vi "Update Control Board.vi"(8 "error in (no error)":errorcluster, 9 "PWM Outputs":T3, 10 "LED Outputs":T4, 11 "Control Board VISA Reference In":refnum<visa-resource-name>) -> (0 "error out":errorcluster, 1 "Analog Inputs":T2, 2 "Switch Inputs":T1, 3 "Control Board VISA Reference Out":refnum<visa-resource-name>, 4 "CRC Status":bool)   [LabVIEW 2013]
uses:
  LED_Output_TypeDef.ctl
  PWM_Output_TypeDef.ctl
  Analog_Input_TypeDef.ctl
  Switch_Input_TypeDef.ctl
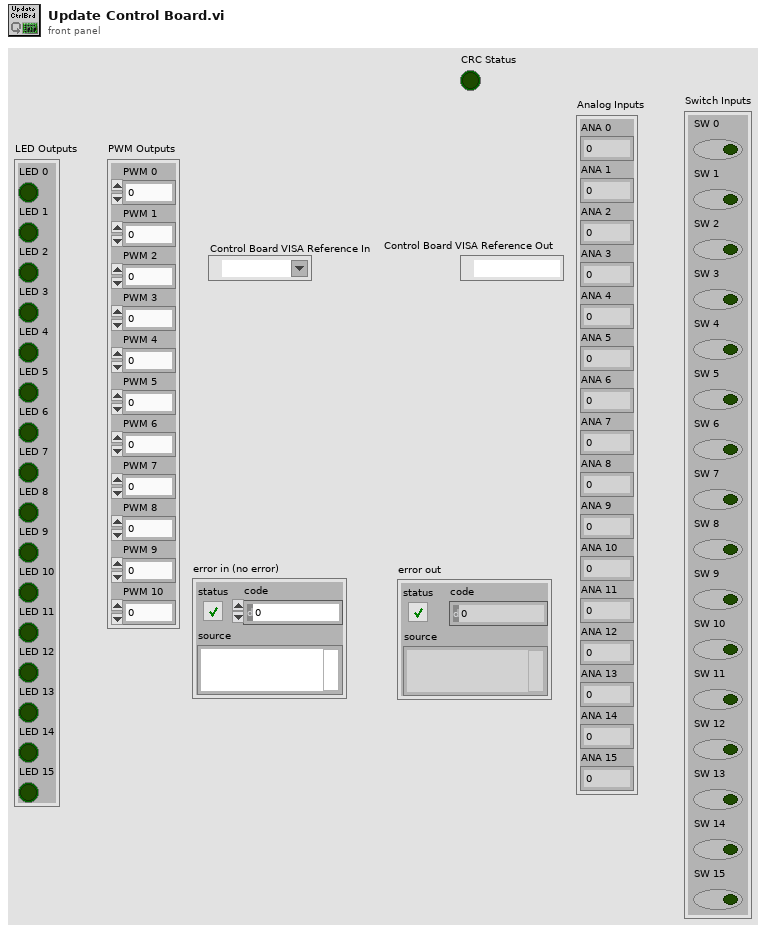
[diagram p1: front panel]
types:
  T1 = typedef "Switch_Input_TypeDef.ctl" = cluster{"SW 0":bool, "SW 1":bool, "SW 2":bool, "SW 3":bool, "SW 4":bool, "SW 5":bool, "SW 6":bool, "SW 7":bool, "SW 8":bool, "SW 9":bool, "SW 10":bool, "SW 11":bool, "SW 12":bool, "SW 13":bool, "SW 14":bool, "SW 15":bool}
  T2 = typedef "Analog_Input_TypeDef.ctl" = cluster{"ANA 0":u8, "ANA 1":u8, "ANA 2":u8, "ANA 3":u8, "ANA 4":u8, "ANA 5":u8, "ANA 6":u8, "ANA 7":u8, "ANA 8":u8, "ANA 9":u8, "ANA 10":u8, "ANA 11":u8, "ANA 12":u8, "ANA 13":u8, "ANA 14":u8, "ANA 15":u8}
  T3 = typedef "PWM_Output_TypeDef.ctl" = cluster{"PWM 0":u8, "PWM 1":u8, "PWM 2":u8, "PWM 3":u8, "PWM 4":u8, "PWM 5":u8, "PWM 6":u8, "PWM 7":u8, "PWM 8":u8, "PWM 9":u8, "PWM 10":u8}
  T4 = typedef "LED_Output_TypeDef.ctl" = cluster{"LED 0":bool, "LED 1":bool, "LED 2":bool, "LED 3":bool, "LED 4":bool, "LED 5":bool, "LED 6":bool, "LED 7":bool, "LED 8":bool, "LED 9":bool, "LED 10":bool, "LED 11":bool, "LED 12":bool, "LED 13":bool, "LED 14":bool, "LED 15":bool}
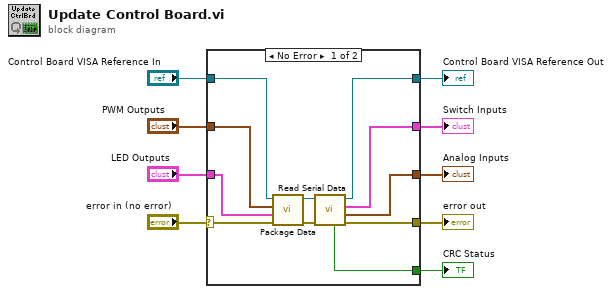
[diagram p0: block diagram]
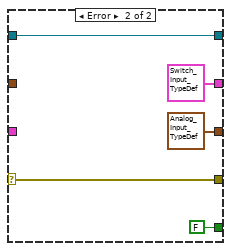
[diagram p2: hidden frame]
diagram:
  n1 = case shown="No Error" "error in (no error)" {
    selector: "error in (no error)" -> [w12 w25]
    tunnel: [w16 w25] -> w8
    tunnel: [w19 T1 {"SW 0"=FALSE, "SW 1"=FALSE, "SW 2"=FALSE, "SW 3"=FALSE, "SW 4"=FALSE, "SW 5"=FALSE, "SW 6"=FALSE, "SW 7"=FALSE, "SW 8"=FALSE, "SW 9"=FALSE, "SW 10"=FALSE, "SW 11"=FALSE, "SW 12"=FALSE, "SW 13"=FALSE, "SW 14"=FALSE, "SW 15"=FALSE} ("Switch Inputs")] -> w7
    tunnel: [w18 T2 {"ANA 0"=0, "ANA 1"=0, "ANA 2"=0, "ANA 3"=0, "ANA 4"=0, "ANA 5"=0, "ANA 6"=0, "ANA 7"=0, "ANA 8"=0, "ANA 9"=0, "ANA 10"=0, "ANA 11"=0, "ANA 12"=0, "ANA 13"=0, "ANA 14"=0, "ANA 15"=0} ("Analog Inputs")] -> w6
    tunnel: "PWM Outputs" -> [w20 _]
    tunnel: "LED Outputs" -> [w17 _]
    tunnel: "Control Board VISA Reference In" -> [w11 w22]
    tunnel: [w15 w22] -> w3
    tunnel: [w10 FALSE ("CRC Status")] -> w1
    frame No Error {
      n2 = call "Package Data.vi"("error in (no error)"=w12, "LED Outputs"=w17, "PWM Outputs"=w20, "VISA resource name in"=w11) -> ("error out"=w13:errorcluster, "VISA resource name out"=w14:refnum<visa-resource-name>)  [unwired: 6 in]
      n3 = call "Read Serial Data.vi"("error in (no error)"=w13, "VISA Refnum in"=w14) -> ("error out"=w16:errorcluster, "Analog Inputs"=w18:T2, "Switch Inputs"=w19:T1, "VISA Refnum out"=w15:refnum<visa-resource-name>, "CRC Status"=w10:bool)  [unwired: 5 in]
    }
    frame Error {
    }
  }
  "Control Board VISA Reference Out" <- w3
  "Switch Inputs" <- w7
  "error out" <- w8
  "Analog Inputs" <- w6
  "CRC Status" <- w1
